vi "setUp.vi"(8 "error in (no error)":errorcluster, 11 "reference in":refnum<class "Create New Assert Tester.lvclass">) -> (0 "error out":errorcluster, 3 "reference out":refnum<class "Create New Assert Tester.lvclass">)   [LabVIEW 2017, in "Create New Assert Tester.lvclass"]
doc: "setUp runs prior to the test method during test execution. Use this method to initialize any object data required by your tests."
uses:
  Create New Assert Tester.lvclass
  C:/Program Files (x86)/National Instruments/LabVIEW 2017/vi.lib/addons/_JKI Toolkits/VI Tester/TestCase.llb/TestCase.lvclass
  Create New Assert Tester.lvclass/Create New Assert Tester.ctl
  <vilib>/addons/_JKI Toolkits/VI Tester/TestCase.llb/TestCase.lvclass
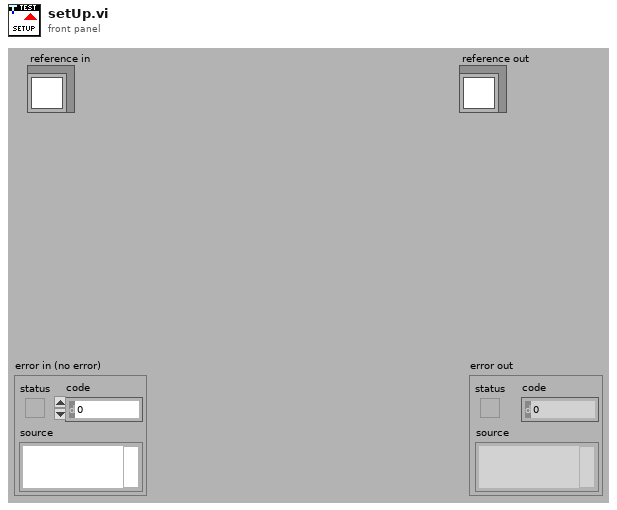
[diagram p1: front panel]
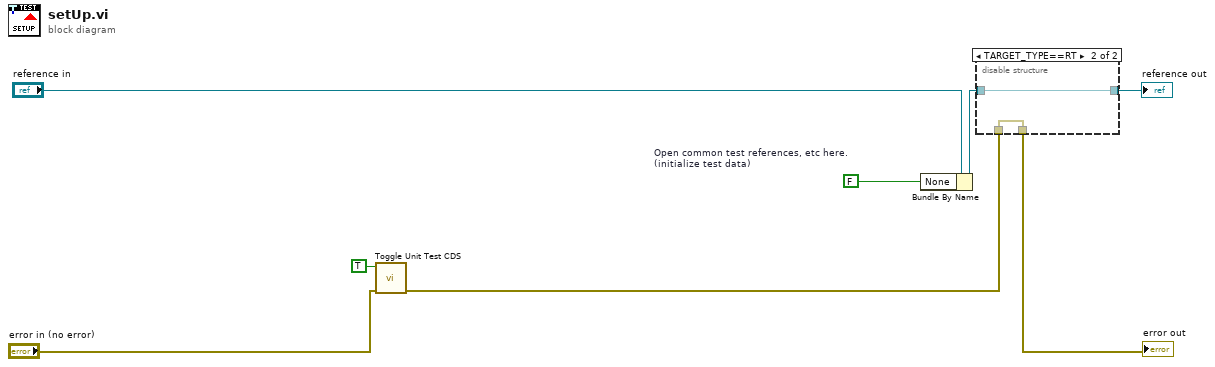
[diagram p0: block diagram]
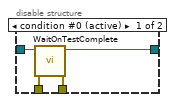
[diagram p2: hidden frame]
diagram:
  w4 = FALSE  # Open common test references, etc here. (initialize test data)
  n1 = call "Toggle Unit Test CDS.vi"("error in (no error)"="error in (no error)", "Requested State"=TRUE) -> ("error out"=w1:errorcluster)  [unwired: 9 in]
  n2 = Bundle By Name(cluster="reference in", "None"=w4) -> (w5:refnum<class "Create New Assert Tester.lvclass">)
  n3 = disable-structure shown="TARGET_TYPE==RT" {
    disable-tunnel: w1 -> [w12 w13]
    disable-tunnel: [w11 w13] -> w8
    disable-tunnel: [w10 w14] -> w6
    disable-tunnel: w5 -> [w9 w14]
    frame condition #0 (active) {
      n4 = call <vilib>:"WaitOnTestComplete.vi"("error in (no error)"=w12, "TestCase in"=w9) -> ("error out"=w11:errorcluster, "TestCase out"=w10:refnum<class "Create New Assert Tester.lvclass">)  [unwired: 8 in]
    }
    frame condition #1 {
    }
  }
  "error out" <- w8
  "reference out" <- w6
